vi "Set Motor Coefficients.vi"(8 "error in (no error)":errorcluster, 10 "Servo Drive and  Motor Paras":T1={"Encoder Output Pulses"=900.0, "Gear Ratio(Numerator)"=1000.0, "Gear Ratio(Denominator)"=1.0, "Reduction Ratio"=1.0} {"Gear Ratio(Denominator)" format="%#_10g"}, 11 "SGDV_Ctrl_Class in":refnum<class "SGDV Motor.lvclass">) -> (0 "error out":errorcluster, 3 "SGDV_Ctrl_Class out":refnum<class "SGDV Motor.lvclass">)   [LabVIEW 2013, in "SGDV_Ctrl_v13_lib.lvlib" / "SGDV Motor.lvclass"]
uses:
  SGDV Motor.lvclass
  Controls and General VIs/Servo Drive and  Motor Paras.ctl
  Controls and General VIs/Motor Coefficients.ctl
  SGDV Motor.lvclass/SGDV Motor.ctl
  SGDV_Ctrl_v13_lib.lvlib
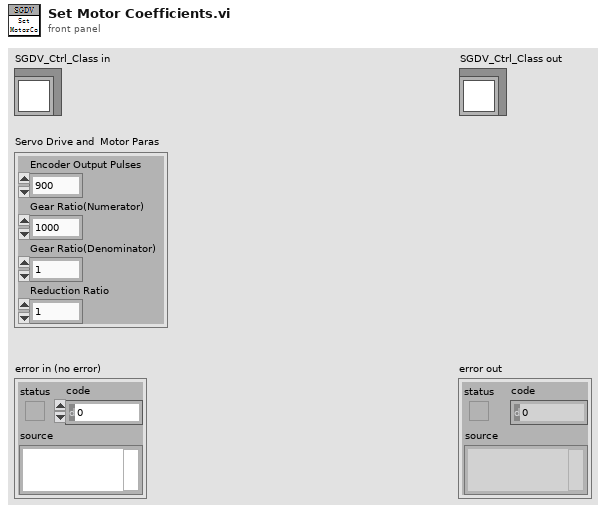
[diagram p1: front panel]
types:
  T1 = typedef "SGDV_Ctrl_v13_lib.lvlib/Servo Drive and  Motor Paras.ctl" = cluster{"Encoder Output Pulses":dbl, "Gear Ratio(Numerator)":dbl, "Gear Ratio(Denominator)":dbl, "Reduction Ratio":dbl}
  T2 = typedef "SGDV_Ctrl_v13_lib.lvlib/Motor Coefficients.ctl" = cluster{"Vel-Coefficient":dbl, "Enc-Coefficient":dbl, "Reduction-Ratio":dbl}
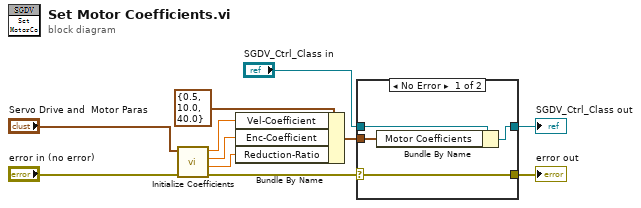
[diagram p0: block diagram]
diagram:
  n1 = call "Initialize Coefficients.vi"("error in (no error)"="error in (no error)", "Servo Drive and  Motor Paras"="Servo Drive and  Motor Paras") -> ("error out"=w2:errorcluster, "Reduction Ratio"=w3:dbl, "Enc-Coefficient"=w4:dbl, "Vel-Coefficient"=w5:dbl)  [unwired: 6 in]
  n2 = Bundle By Name(cluster=T2 {"Vel-Coefficient"=0.5, "Enc-Coefficient"=10.0, "Reduction-Ratio"=40.0} ("Motor Coefficients"), "Vel-Coefficient"=w5, "Enc-Coefficient"=w4, "Reduction-Ratio"=w3) -> (w1:T2)
  n3 = case shown="No Error" w2 {
    selector: w2 -> [w15 w16]
    tunnel: [w15 w16] -> w11
    tunnel: [w13 w17] -> w9
    tunnel: "SGDV_Ctrl_Class in" -> [w14 w17]
    tunnel: w1 -> [w12 _]
    frame No Error {
      n4 = Bundle By Name(cluster=w14, "Motor Coefficients"=w12) -> (w13:refnum<class "SGDV Motor.lvclass">)
    }
    frame Error {
    }
  }
  "error out" <- w11
  "SGDV_Ctrl_Class out" <- w9
